vi "DAQmx USB6008.vi"() -> (0 "Temperature data":dbl)   [LabVIEW 2023]
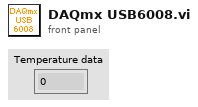
[diagram p1: front panel]
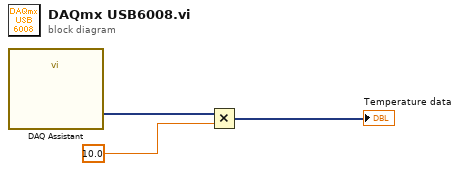
[diagram p0: block diagram]
diagram:
  n1 = call "DAQ Assistant"() -> ("data"=w3:dynamicdata)  [unwired: 17 in, 2 out]
  n2 = Multiply(x=w3, y=10.0) -> (x*y=→"Temperature data":dynamicdata)
